vi "main_loop_calculation.vi"(8 "PG Data":waveform(dbl)[](array[waveform]), 9 "Offset Parameters":T1={"Liquid Tank\nPressure"=0.0, "Liquid Tank\nTemperature"=0.0, "Separator Pressure"=0.0, "Separator \nTemperature"=0.0, "Liquid Inlet\nPressure"=0.0, "Liquid Inlet\nTemperature "=0.0, "Vapor Tank\nPressure "=0.0, "Vapor Tank\nTemperature "=0.0, "Vapor Inlet\nPressure"=0.0, "Vapor Inlet \nTemperature"=0.0, "Test Section\nPressure"=0.0, "Test Section\nTemperature"=0.0, "Upper Dev Section\nPressure"=0.0, "Upper Dev Section\nTemperature"=0.0, "Lower Dev Section\nPressure"=0.0, "PG Inlet-Mixing Tee Pressure"=0.0, "Vapor Line dP"=0.0, "Atmospheric Pressure [Pa]"=101325.0}, 10 "Session Start Time":timestamp, 11 "DAQ Data":waveform(dbl)[](array[waveform])) -> (0 "Pressure/Temperature/Mixture Properties":T4, 1 "Liquid Flow Data":T2, 2 "Vapor Flow Data":T3, 4 "Converted Data":dbl[][](array[numeric]), 6 "Raw Data":dbl[][](array[numeric]))   [LabVIEW 2017]
uses:
  pressure_temp_mixture.ctl
  offset_parameters.ctl
  <vilib>/Waveform/WDTOps.llb/WDT Get Waveform Time Array DBL.vi
  Sensor Translation/Pressure Transducers/Omega/omega_px209_060a5v.vi
  Sensor Translation/Pressure Transducers/Setra/setra_2301_002PD_2F2D.vi
  Sensor Translation/Pressure Transducers/Omega/omega_px303_050a5v.vi
  Sensor Translation/MicroFlow Transducers/microflow_density.vi
  Sensor Translation/MicroFlow Transducers/microflow_mass_flow.vi
  Sensor Translation/pressure_unit_converter.vi
  Sensor Translation/sensor_translation.lvlib
panel:
  out "Separator Temp":dbl
  out "Liquid Inlet T":dbl
  out "Vapor Inlet T Sat":dbl
  # "Saturation\nPressure [Pa]"
  # "Saturation\nTemperature [C]"
  # "Pressure [Pa]"
  # "Temperature [C]"
  # "Liquid Tank"
  # "Separator"
  # "Liquid Inlet"
  # "Vapor Tank"
  # "Vapor Inlet"
  # "Test Section"
  # "Upper Dev Section"
  # "Lower Dev Section"
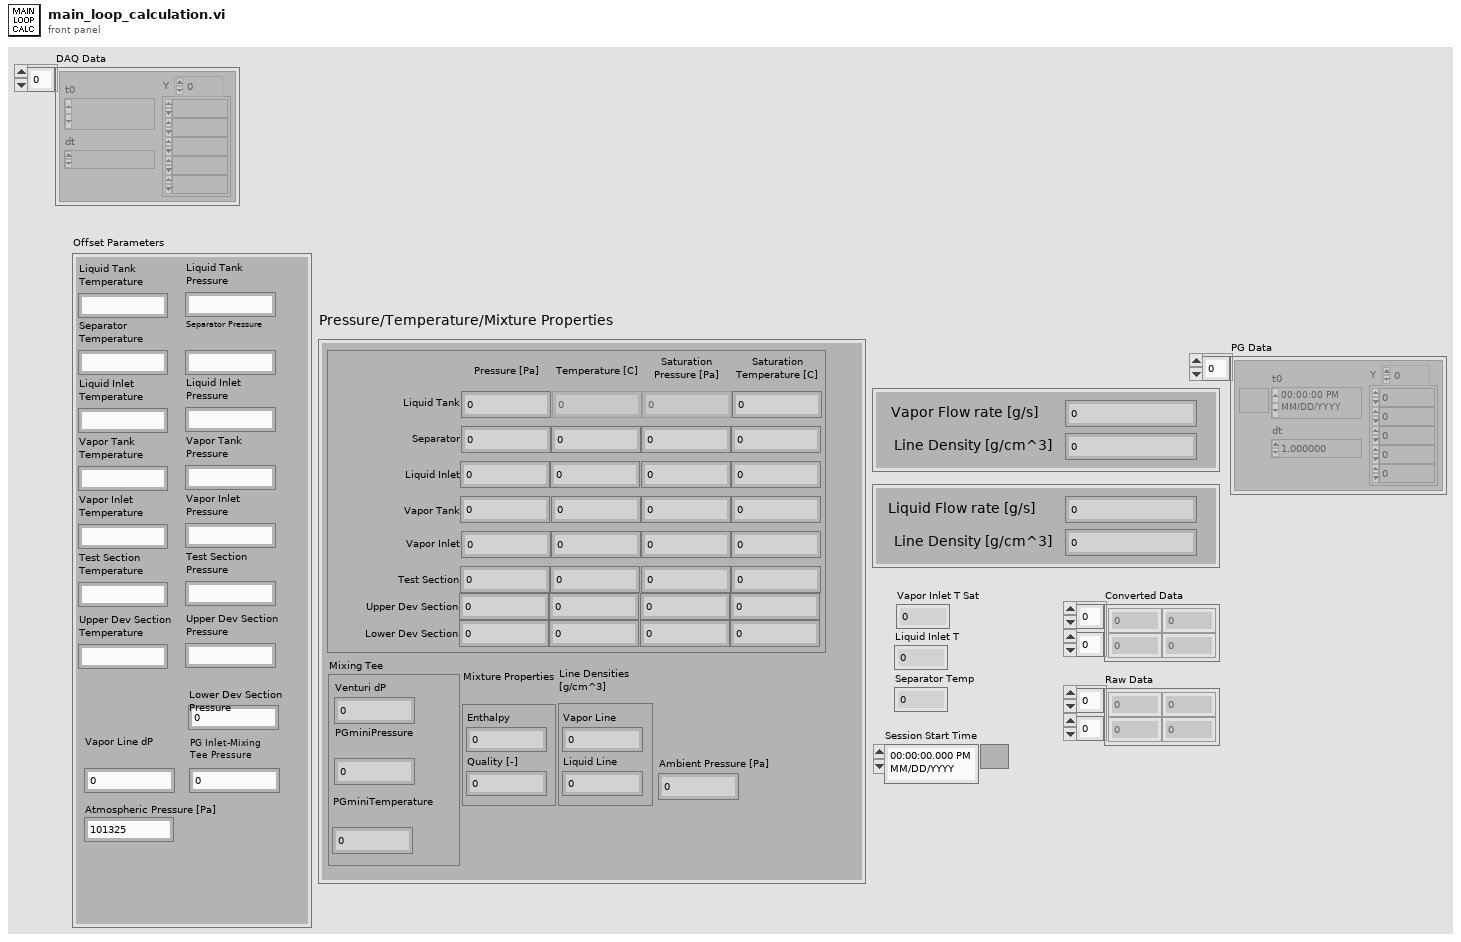
[diagram p1: front panel]
types:
  T1 = typedef "offset_parameters.ctl" = cluster{"Liquid Tank\nPressure":dbl, "Liquid Tank\nTemperature":dbl, "Separator Pressure":dbl, "Separator \nTemperature":dbl, "Liquid Inlet\nPressure":dbl, "Liquid Inlet\nTemperature ":dbl, "Vapor Tank\nPressure ":dbl, "Vapor Tank\nTemperature ":dbl, "Vapor Inlet\nPressure":dbl, "Vapor Inlet \nTemperature":dbl, "Test Section\nPressure":dbl, "Test Section\nTemperature":dbl, "Upper Dev Section\nPressure":dbl, "Upper Dev Section\nTemperature":dbl, "Lower Dev Section\nPressure":dbl, "PG Inlet-Mixing Tee Pressure":dbl, "Vapor Line dP":dbl, "Atmospheric Pressure [Pa]":dbl}
  T2 = cluster{"Liquid Flow rate [g/s]":dbl, "Line Density [g/cm^3]":dbl}
  T3 = cluster{"Vapor Flow rate [g/s]":dbl, "Line Density [g/cm^3]":dbl}
  T4 = typedef "pressure_temp_mixture.ctl" = cluster{"Line Densities\n[g/cm^3]":cluster{"Vapor Line":dbl, "Liquid Line":dbl}, "Mixture Properties":cluster{"Enthalpy":dbl, "Quality [-]":dbl}, "Component PTs":cluster{"Liquid Tank P":dbl, "Liquid Tank T":dbl, "Liquid Tank Sat P":dbl, "Liquid Tank Sat T":dbl, "Separator P":dbl, "Separator T":dbl, "Separator Sat P":dbl, "Separator Sat T":dbl, "Liquid Inlet P":dbl, "Liquid Inlet T":dbl, "Liquid Inlet Sat P":dbl, "Liquid Inlet Sat T":dbl, "Vapor Tank P":dbl, "Vapor Tank T":dbl, "Vapor Tank Sat P":dbl, "Vapor Tank Sat T":dbl, "Vapor Inlet P":dbl, "Vapor Inlet T":dbl, "Vapor Inlet Sat P":dbl, "Vapor Inlet Sat T":dbl, "Test Section P":dbl, "Test Section T":dbl, "Test Section Sat P":dbl, "Test Section Sat T":dbl, "Upper Dev Section P":dbl, "Upper Dev Section T":dbl, "Upper Dev Section Sat P":dbl, "Upper Dev Section Sat T":dbl, "Lower Dev Section P":dbl, "Lower Dev Section T":dbl, "Lower Dev Section Sat P":dbl, "Lower Dev Section Sat T":dbl}, "Ambient Pressure [Pa]":dbl, "Mixing Tee":cluster{"Venturi dP":dbl, "PGminiPressure":dbl, "PGminiTemperature":dbl}}
  T5 = cluster{"Offset Average":dbl, "Offset Average":dbl, "Offset Average":dbl}
  T6 = cluster{"Rounded Value":dbl, "Rounded Value":dbl}
  T7 = cluster{"mixture enthalpy":dbl, "Quality [-]":dbl}
  T8 = cluster{"array[0]":dbl, "array[1]":dbl, "array[2]":dbl, "array[3]":dbl, "array[4]":dbl, "array[5]":dbl, "array[6]":dbl, "array[7]":dbl, "array[8]":dbl, "array[9]":dbl, "array[10]":dbl, "array[11]":dbl, "array[12]":dbl, "array[13]":dbl, "array[14]":dbl, "array[15]":dbl, "array[16]":dbl, "array[17]":dbl, "array[18]":dbl, "array[19]":dbl, "array[20]":dbl, "array[21]":dbl, "array[22]":dbl, "array[23]":dbl, "array[24]":dbl, "array[25]":dbl, "array[26]":dbl, "array[27]":dbl, "array[28]":dbl, "array[29]":dbl, "array[30]":dbl, "array[31]":dbl}
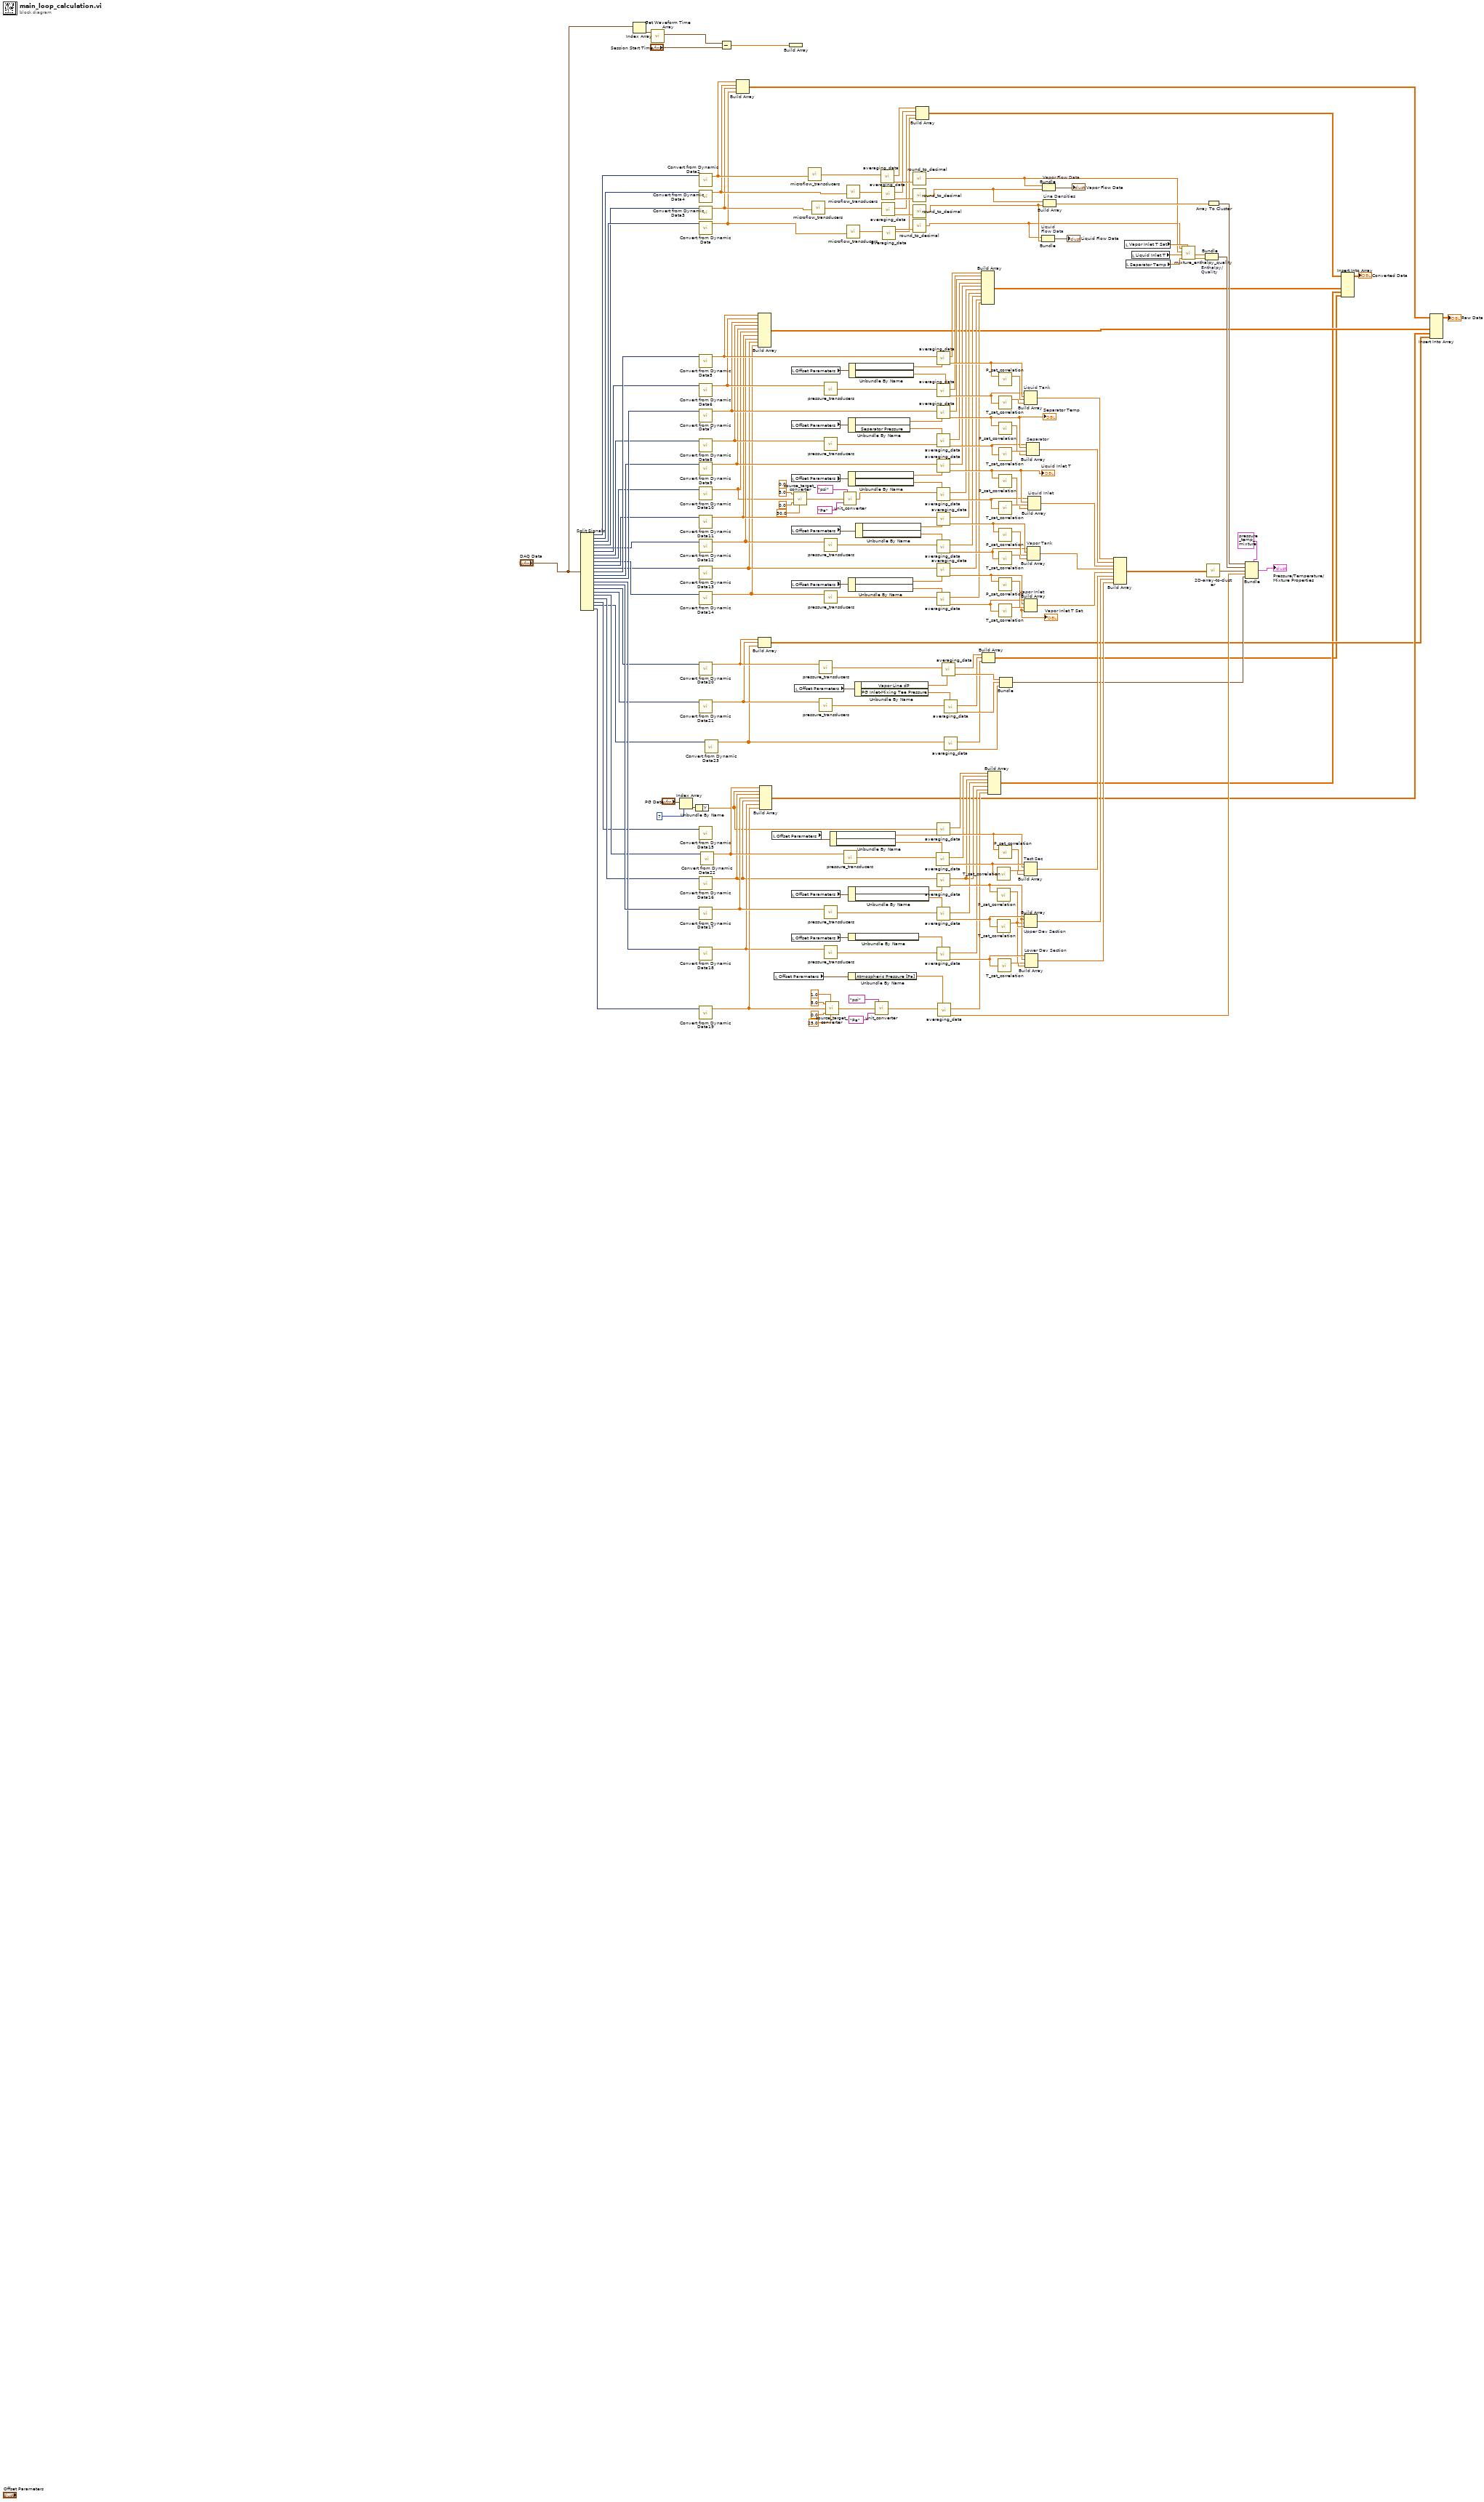
[diagram p0: block diagram]
diagram:
  (unwired) 0.0 ("Source Low")
  n1 = Split Signals("DAQ Data") -> (w183:dynamicdata, w177:dynamicdata, w206:dynamicdata, w205:dynamicdata, w146:dynamicdata, w166:dynamicdata, w160:dynamicdata, w152:dynamicdata, w140:dynamicdata, w148:dynamicdata, w125:dynamicdata, w168:dynamicdata, w155:dynamicdata, w161:dynamicdata, w127:dynamicdata, w128:dynamicdata, w92:dynamicdata, w91:dynamicdata, w4:dynamicdata, w3:dynamicdata, w2:dynamicdata, w1:dynamicdata, w9:dynamicdata)  [unwired: 23 in]
  n2 = Index Array(array="DAQ Data") -> (element=w93:waveform(dbl))  [unwired: 1 in]
  n3 = call-poly <vilib>:"Get Waveform Time Array.vi"("waveform in"=w93) -> ("X array"=w40:timestamp[])  [unwired: 9 in, 1 out]
  n4 = Index Array(array="PG Data", index=7) -> (element=w11:waveform(dbl))
  n5 = Unbundle By Name(w11) -> ("Y"=w10:dbl[])
  n6 = call "Convert from Dynamic Data2"("Dynamic Data Type"=w183) -> ("Array"=w82:dbl[])  [unwired: 3 in]
  n7 = call "Convert from Dynamic Data4"("Dynamic Data Type"=w177) -> ("Array"=w81:dbl[])  [unwired: 3 in]
  n8 = call "Convert from Dynamic Data3"("Dynamic Data Type"=w205) -> ("Array"=w80:dbl[])  [unwired: 3 in]
  n9 = call "Convert from Dynamic Data"("Dynamic Data Type"=w206) -> ("Array"=w79:dbl[])  [unwired: 3 in]
  n10 = call "Convert from Dynamic Data5"("Dynamic Data Type"=w168) -> ("Array"=w78:dbl[])  [unwired: 3 in]
  n11 = call "Convert from Dynamic Data6"("Dynamic Data Type"=w166) -> ("Array"=w77:dbl[])  [unwired: 3 in]
  n12 = call "Convert from Dynamic Data7"("Dynamic Data Type"=w161) -> ("Array"=w76:dbl[])  [unwired: 3 in]
  n13 = call "Convert from Dynamic Data8"("Dynamic Data Type"=w160) -> ("Array"=w75:dbl[])  [unwired: 3 in]
  n14 = call "Convert from Dynamic Data9"("Dynamic Data Type"=w155) -> ("Array"=w74:dbl[])  [unwired: 3 in]
  n15 = call "Convert from Dynamic Data10"("Dynamic Data Type"=w152) -> ("Array"=w32:dbl[])  [unwired: 3 in]
  n16 = call "Convert from Dynamic Data11"("Dynamic Data Type"=w148) -> ("Array"=w73:dbl[])  [unwired: 3 in]
  n17 = call "Convert from Dynamic Data12"("Dynamic Data Type"=w146) -> ("Array"=w72:dbl[])  [unwired: 3 in]
  n18 = call "Convert from Dynamic Data13"("Dynamic Data Type"=w125) -> ("Array"=w71:dbl[])  [unwired: 3 in]
  n19 = call "Convert from Dynamic Data14"("Dynamic Data Type"=w140) -> ("Array"=w70:dbl[])  [unwired: 3 in]
  n20 = call "Convert from Dynamic Data20"("Dynamic Data Type"=w92) -> ("Array"=w68:dbl[])  [unwired: 3 in]
  n21 = call "Convert from Dynamic Data21"("Dynamic Data Type"=w91) -> ("Array"=w67:dbl[])  [unwired: 3 in]
  n22 = call "Convert from Dynamic Data15"("Dynamic Data Type"=w2) -> ()  [unwired: 3 in, 1 out]
  n23 = call "Convert from Dynamic Data16"("Dynamic Data Type"=w3) -> ("Array"=w41:dbl[])  [unwired: 3 in]
  n24 = call "Convert from Dynamic Data17"("Dynamic Data Type"=w128) -> ("Array"=w69:dbl[])  [unwired: 3 in]
  n25 = call "Convert from Dynamic Data18"("Dynamic Data Type"=w127) -> ("Array"=w42:dbl[])  [unwired: 3 in]
  n26 = call "Convert from Dynamic Data19"("Dynamic Data Type"=w9) -> ("Array"=w43:dbl[])  [unwired: 3 in]
  n27 = call "Convert from Dynamic Data22"("Dynamic Data Type"=w4) -> ("Array"=w207:dbl[])  [unwired: 3 in]
  n28 = call "Convert from Dynamic Data23"("Dynamic Data Type"=w1) -> ("Array"=w8:dbl[])  [unwired: 3 in]
  n29 = Subtract(x=w40, y="Session Start Time") -> (x-y=w44:dbl[])
  n30 = Build Array(w82, w81, w80, w79) -> (w23:dbl[][])
  n31 = Build Array(w78, w77, w76, w75, w74, w32, w73, w72, w71, w70) -> (w22:dbl[][])
  n32 = Build Array(w68, w67, w8) -> (w20:dbl[][])
  n33 = Build Array(w207, w10, w41, w69, w41, w42, w43) -> (w21:dbl[][])
  n34 = local read "Offset Parameters"() -> (w134:T1)
  n35 = local read "Offset Parameters"() -> (w185:T1)
  n36 = Build Array(w44) -> ()  [unwired: 1 out]
  n37 = local read "Offset Parameters"() -> (w195:T1)
  n38 = local read "Offset Parameters"() -> (w193:T1)
  n39 = local read "Offset Parameters"() -> (w192:T1)
  n40 = local read "Offset Parameters"() -> (w196:T1)
  n41 = local read "Offset Parameters"() -> (w194:T1)
  n42 = local read "Offset Parameters"() -> (w129:T1)
  n43 = local read "Offset Parameters"() -> (w122:T1)
  n44 = call "source_target_converter.vi"("Source High"=5.0, "Source"=w32, "Target Low"=0.0, "Target High"=30.0) -> ("Target"=w35:dbl[])  [unwired: 1 in]
  n45 = local read "Offset Parameters"() -> (w88:T1)
  n46 = call-poly "microflow_transducers.vi"("Source"=w82) -> ("Target"=w109:dbl[])  [unwired: 3 in]
  n47 = call-poly "microflow_transducers.vi"("Source"=w80) -> ("Target"=w110:dbl[])  [unwired: 3 in]
  n48 = call-poly "pressure_transducers.vi"("Source"=w68) -> ("Target"=w90:dbl[])  [unwired: 1 in]
  n49 = call-poly "pressure_transducers.vi"("Source"=w67) -> ("Target"=w89:dbl[])  [unwired: 1 in]
  n50 = call-poly "pressure_transducers.vi"("Source"=w77) -> ("Target"=w163:dbl[])  [unwired: 1 in]
  n51 = call-poly "pressure_transducers.vi"("Source"=w75) -> ("Target"=w153:dbl[])  [unwired: 1 in]
  n52 = call-poly "pressure_transducers.vi"("Source"=w72) -> ("Target"=w145:dbl[])  [unwired: 1 in]
  n53 = call-poly "pressure_transducers.vi"("Source"=w70) -> ("Target"=w138:dbl[])  [unwired: 1 in]
  n54 = call-poly "pressure_transducers.vi"("Source"=w69) -> ("Target"=w132:dbl[])  [unwired: 1 in]
  n55 = call-poly "pressure_transducers.vi"("Source"=w42) -> ("Target"=w126:dbl[])  [unwired: 1 in]
  n56 = call "source_target_converter.vi"("Source High"=5.0, "Source Low"=1.0, "Source"=w43, "Target Low"=0.0, "Target High"=25.0) -> ("Target"=w97:dbl[])
  n57 = Unbundle By Name(w134) -> ("Test Section\nTemperature"=w133:dbl, "Test Section\nPressure"=w15:dbl)
  n58 = call-poly "unit_converter.vi"("Output Unit"="Pa", "Input"=w35, "Input Unit"="psi") -> ("Output"=w31:dbl[])
  n59 = call-poly "pressure_transducers.vi"("Source"=w207) -> ("Target"=w27:dbl[])  [unwired: 1 in]
  n60 = call-poly "microflow_transducers.vi"("Source"=w81) -> ("Target"=w112:dbl[])  [unwired: 3 in]
  n61 = call-poly "microflow_transducers.vi"("Source"=w79) -> ("Target"=w111:dbl[])  [unwired: 3 in]
  n62 = Unbundle By Name(w193) -> ("Separator \nTemperature"=w162:dbl, "Separator Pressure"=w159:dbl)
  n63 = Unbundle By Name(w192) -> ("Liquid Inlet\nTemperature"=w154:dbl, "Liquid Inlet\nPressure"=w151:dbl)
  n64 = Unbundle By Name(w194) -> ("Vapor Inlet \nTemperature"=w141:dbl, "Vapor Inlet\nPressure"=w139:dbl)
  n65 = Unbundle By Name(w129) -> ("Upper Dev Section\nTemperature"=w130:dbl, "Upper Dev Section\nPressure"=w131:dbl)
  n66 = Unbundle By Name(w122) -> ("Lower Dev Section\nPressure"=w121:dbl)
  n67 = Unbundle By Name(w185) -> ("Atmospheric Pressure [Pa]"=w103:dbl)
  n68 = Unbundle By Name(w195) -> ("Liquid Tank\nTemperature"=w167:dbl, "Liquid Tank\nPressure"=w165:dbl)
  n69 = Unbundle By Name(w88) -> ("Vapor Line dP"=w87:dbl, "PG Inlet-Mixing Tee Pressure"=w86:dbl)
  n70 = Unbundle By Name(w196) -> ("Vapor Tank\nTemperature"=w147:dbl, "Vapor Tank\nPressure"=w144:dbl)
  n71 = call-poly "unit_converter.vi"("Output Unit"="Pa", "Input"=w97, "Input Unit"="psi") -> ("Output"=w94:dbl[])
  n72 = call "averaging_data.vi"("Input"=w109) -> ("Offset Average"=w53:dbl, "Input Out"=w47:dbl[])  [unwired: 6 in, 2 out]
  n73 = call "averaging_data.vi"("Input"=w112) -> ("Offset Average"=w52:dbl, "Input Out"=w48:dbl[])  [unwired: 6 in, 2 out]
  n74 = call "averaging_data.vi"("Input"=w110) -> ("Offset Average"=w51:dbl, "Input Out"=w49:dbl[])  [unwired: 6 in, 2 out]
  n75 = call "averaging_data.vi"("Input"=w111) -> ("Input Out"=w50:dbl[], "Average"=w104:dbl)  [unwired: 6 in, 2 out]
  n76 = call "round_to_decimal.vi"("Value to Round"=w53) -> ("Rounded Value"=w108:dbl)  [unwired: 1 in]
  n77 = call "round_to_decimal.vi"("Value to Round"=w52) -> ("Rounded Value"=w107:dbl)  [unwired: 1 in]
  n78 = call "round_to_decimal.vi"("Value to Round"=w51) -> ("Rounded Value"=w106:dbl)  [unwired: 1 in]
  n79 = call "round_to_decimal.vi"("Value to Round"=w104) -> ("Rounded Value"=w105:dbl)  [unwired: 1 in]
  n80 = Build Array(w47, w48, w49, w50) -> (w19:dbl[][])
  n81 = call "averaging_data.vi"("Offset"=w15, "Input"=w27) -> ("Offset Average"=w208:dbl, "Input Out"=w24:dbl[])  [unwired: 5 in, 2 out]
  n82 = call "averaging_data.vi"("Offset"=w167, "Input"=w78) -> ("Offset Average"=w169:dbl, "Input Out"=w65:dbl[])  [unwired: 5 in, 2 out]
  n83 = call "averaging_data.vi"("Offset"=w165, "Input"=w163) -> ("Offset Average"=w164:dbl, "Input Out"=w64:dbl[])  [unwired: 5 in, 2 out]
  n84 = call "averaging_data.vi"("Offset"=w162, "Input"=w76) -> ("Offset Average"=w158:dbl, "Input Out"=w63:dbl[])  [unwired: 5 in, 2 out]
  "Separator Temp" <- w158
  n85 = call "averaging_data.vi"("Offset"=w159, "Input"=w153) -> ("Offset Average"=w156:dbl, "Input Out"=w62:dbl[])  [unwired: 5 in, 2 out]
  n86 = call "averaging_data.vi"("Offset"=w154, "Input"=w74) -> ("Offset Average"=w150:dbl, "Input Out"=w61:dbl[])  [unwired: 5 in, 2 out]
  "Liquid Inlet T" <- w150
  n87 = call "averaging_data.vi"("Offset"=w151, "Input"=w31) -> ("Offset Average"=w149:dbl, "Input Out"=w60:dbl[])  [unwired: 5 in, 2 out]
  n88 = call "averaging_data.vi"("Offset"=w147, "Input"=w73) -> ("Offset Average"=w143:dbl, "Input Out"=w59:dbl[])  [unwired: 5 in, 2 out]
  n89 = call "averaging_data.vi"("Offset"=w144, "Input"=w145) -> ("Offset Average"=w142:dbl, "Input Out"=w58:dbl[])  [unwired: 5 in, 2 out]
  n90 = call "averaging_data.vi"("Offset"=w141, "Input"=w71) -> ("Offset Average"=w135:dbl, "Input Out"=w57:dbl[])  [unwired: 5 in, 2 out]
  n91 = call "averaging_data.vi"("Offset"=w139, "Input"=w138) -> ("Offset Average"=w137:dbl, "Input Out"=w56:dbl[])  [unwired: 5 in, 2 out]
  n92 = call "averaging_data.vi"("Offset"=w133, "Input"=w10) -> ("Offset Average"=w123:dbl, "Input Out"=w25:dbl[])  [unwired: 5 in, 2 out]
  n93 = call "averaging_data.vi"("Offset"=w130, "Input"=w41) -> ("Offset Average"=w114:dbl, "Input Out"=w28:dbl[])  [unwired: 5 in, 2 out]
  n94 = call "averaging_data.vi"("Offset"=w131, "Input"=w132) -> ("Offset Average"=w120:dbl, "Input Out"=w46:dbl[])  [unwired: 5 in, 2 out]
  n95 = call "averaging_data.vi"("Offset"=w121, "Input"=w126) -> ("Offset Average"=w117:dbl, "Input Out"=w29:dbl[])  [unwired: 5 in, 2 out]
  n96 = call "averaging_data.vi"("Offset"=w103, "Input"=w94) -> ("Offset Average"=w98:dbl, "Input Out"=w30:dbl[])  [unwired: 5 in, 2 out]
  n97 = call "averaging_data.vi"("Offset"=w87, "Input"=w90) -> ("Offset Average"=w85:dbl, "Input Out"=w55:dbl[])  [unwired: 5 in, 2 out]
  n98 = call "averaging_data.vi"("Input"=w8) -> ("Offset Average"=w6:dbl, "Input Out"=w7:dbl[])  [unwired: 6 in, 2 out]
  n99 = call "averaging_data.vi"("Offset"=w86, "Input"=w89) -> ("Offset Average"=w84:dbl, "Input Out"=w54:dbl[])  [unwired: 5 in, 2 out]
  n100 = Build Array(w65, w64, w63, w62, w61, w60, w59, w58, w57, w56) -> (w18:dbl[][])
  n101 = Build Array(w55, w54, w7) -> (w16:dbl[][])
  n102 = Build Array(w25, w24, w28, w46, w28, w29, w30) -> (w17:dbl[][])
  n103 = call "T_sat_correlation.vi"("P [Pa]"=w208) -> ("T Sat [C]"=w26:dbl)  [unwired: 1 out]
  n104 = call "P_sat_correlation.vi"("Temperature[C]"=w114) -> ("P Sat[Pa]"=w113:dbl)  [unwired: 1 in, 1 out]
  n105 = call "T_sat_correlation.vi"("P [Pa]"=w120) -> ("T Sat [C]"=w119:dbl)  [unwired: 1 out]
  n106 = call "T_sat_correlation.vi"("P [Pa]"=w117) -> ("T Sat [C]"=w118:dbl)  [unwired: 1 out]
  n107 = call "P_sat_correlation.vi"("Temperature[C]"=w169) -> ("P Sat[Pa]"=w204:dbl)  [unwired: 1 in, 1 out]
  n108 = call "T_sat_correlation.vi"("P [Pa]"=w164) -> ("T Sat [C]"=w203:dbl)  [unwired: 1 out]
  n109 = call "P_sat_correlation.vi"("Temperature[C]"=w158) -> ("P Sat[Pa]"=w197:dbl)  [unwired: 1 in, 1 out]
  n110 = call "T_sat_correlation.vi"("P [Pa]"=w156) -> ("T Sat [C]"=w157:dbl)  [unwired: 1 out]
  n111 = call "P_sat_correlation.vi"("Temperature[C]"=w150) -> ("P Sat[Pa]"=w199:dbl)  [unwired: 1 in, 1 out]
  n112 = call "T_sat_correlation.vi"("P [Pa]"=w149) -> ("T Sat [C]"=w198:dbl)  [unwired: 1 out]
  n113 = call "P_sat_correlation.vi"("Temperature[C]"=w143) -> ("P Sat[Pa]"=w201:dbl)  [unwired: 1 in, 1 out]
  n114 = call "T_sat_correlation.vi"("P [Pa]"=w142) -> ("T Sat [C]"=w202:dbl)  [unwired: 1 out]
  n115 = call "P_sat_correlation.vi"("Temperature[C]"=w135) -> ("P Sat[Pa]"=w200:dbl)  [unwired: 1 in, 1 out]
  n116 = call "T_sat_correlation.vi"("P [Pa]"=w137) -> ("T Sat [C]"=w136:dbl)  [unwired: 1 out]
  "Vapor Inlet T Sat" <- w136
  n117 = call "P_sat_correlation.vi"("Temperature[C]"=w123) -> ("P Sat[Pa]"=w124:dbl)  [unwired: 1 in, 1 out]
  n118 = Bundle("Offset Average"=w85, "Offset Average"=w84, "Offset Average"=w6) -> (w83:T5)  [unwired: 1 in]
  n119 = Build Array "Liquid Tank"(w164, w169, w204, w203) -> (w187:dbl[])
  n120 = Build Array "Vapor Inlet"(w137, w135, w200, w136) -> (w189:dbl[])
  n121 = Build Array "Test Sec"(w208, w123, w124, w26) -> (w188:dbl[])
  n122 = Build Array "Upper Dev Section"(w120, w114, w113, w119) -> (w116:dbl[])
  n123 = Build Array "Lower Dev Section"(w117, w114, w113, w118) -> (w115:dbl[])
  n124 = Build Array "Separator"(w156, w158, w197, w157) -> (w186:dbl[])
  n125 = Build Array "Vapor Tank"(w142, w143, w201, w202) -> (w190:dbl[])
  n126 = Build Array "Liquid Inlet"(w149, w150, w199, w198) -> (w191:dbl[])
  n127 = Bundle "Liquid\nFlow Data"("Rounded Value"=w105, "Rounded Value"=w106) -> (→"Liquid Flow Data":T6)  [unwired: 1 in]
  n128 = Bundle "Vapor Flow Data"("Rounded Value"=w108, "Rounded Value"=w107) -> (→"Vapor Flow Data":T6)  [unwired: 1 in]
  n129 = Build Array "Line Densities"(w107, w106) -> (w180:dbl[])
  n130 = Build Array(w187, w186, w191, w190, w189, w188, w116, w115) -> (w184:dbl[][])
  n131 = local read "Vapor Inlet T Sat"() -> (w171:dbl)
  n132 = local read "Separator Temp"() -> (w173:dbl)
  n133 = local read "Liquid Inlet T"() -> (w172:dbl)
  n134 = call "mixture_enthalpy_quality.vi"("Vapor Inlet Pressure [Pa]"=w171, "Separator Temp [C]"=w173, "Liquid Inlet Temp [C]"=w172, "Vapor Flow Rate [g/s]"=w108, "Liquid Flow Rate [g/s]"=w105) -> ("Quality [-]"=w181:dbl, "mixture enthalpy"=w182:dbl)  [unwired: 2 out]
  n135 = Bundle "Enthalpy/\nQuality"("mixture enthalpy"=w182, "Quality [-]"=w181) -> (w175:T7)  [unwired: 1 in]
  n136 = call "2D-array-to-cluster.vi"("2D Array"=w184) -> ("Cluster"=w176:T8)
  n137 = Array To Cluster(array=w180) -> (cluster=w174:cluster{"[0]":dbl, "[1]":dbl})
  n138 = Bundle(cluster=T4 {"Line Densities\n[g/cm^3]"={"Vapor Line"=0.0, "Liquid Line"=0.0}, "Mixture Properties"={"Enthalpy"=0.0, "Quality [-]"=0.0}, "Component PTs"={"Liquid Tank P"=0.0, "Liquid Tank T"=0.0, "Liquid Tank Sat P"=0.0, "Liquid Tank Sat T"=0.0, "Separator P"=0.0, "Separator T"=0.0, "Separator Sat P"=0.0, "Separator Sat T"=0.0, "Liquid Inlet P"=0.0, "Liquid Inlet T"=0.0, "Liquid Inlet Sat P"=0.0, "Liquid Inlet Sat T"=0.0, "Vapor Tank P"=0.0, "Vapor Tank T"=0.0, "Vapor Tank Sat P"=0.0, "Vapor Tank Sat T"=0.0, "Vapor Inlet P"=0.0, "Vapor Inlet T"=0.0, "Vapor Inlet Sat P"=0.0, "Vapor Inlet Sat T"=0.0, "Test Section P"=0.0, "Test Section T"=0.0, "Test Section Sat P"=0.0, "Test Section Sat T"=0.0, "Upper Dev Section P"=0.0, "Upper Dev Section T"=0.0, "Upper Dev Section Sat P"=0.0, "Upper Dev Section Sat T"=0.0, "Lower Dev Section P"=0.0, "Lower Dev Section T"=0.0, "Lower Dev Section Sat P"=0.0, "Lower Dev Section Sat T"=0.0}, "Ambient Pressure [Pa]"=0.0, "Mixing Tee"={"Venturi dP"=0.0, "PGminiPressure"=0.0, "PGminiTemperature"=0.0}} ("Pressure/Temperature/Mixture Properties"), "Line Densities\n[g/cm^3]"=w174, "Mixture Properties"=w175, "Component PTs"=w176, "Ambient Pressure [Pa]"=w98, "Mixing Tee"=w83) -> (→"Pressure/Temperature/Mixture Properties":T4)
  n139 = Insert Into Array(array=w19, new element #1=w18, new element #2=w17, new element #3=w16) -> (→"Converted Data":dbl[][])  [unwired: 2 in]
  n140 = Insert Into Array(array=w23, new element #1=w22, new element #2=w21, new element #3=w20) -> (→"Raw Data":dbl[][])  [unwired: 2 in]
